vi "Gyro Vision Update.vi"() -> ()   [LabVIEW 2013]
uses:
  Robot Global Data.vi
  <vilib>/Rock Robotics/WPI/Gyro/WPI_GyroRefNum Registry Get.vi
  <vilib>/Rock Robotics/WPI/Gyro/WPI_GyroGetAngle.vi
panel:
  out "Success":bool
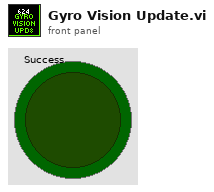
[diagram p1: front panel]
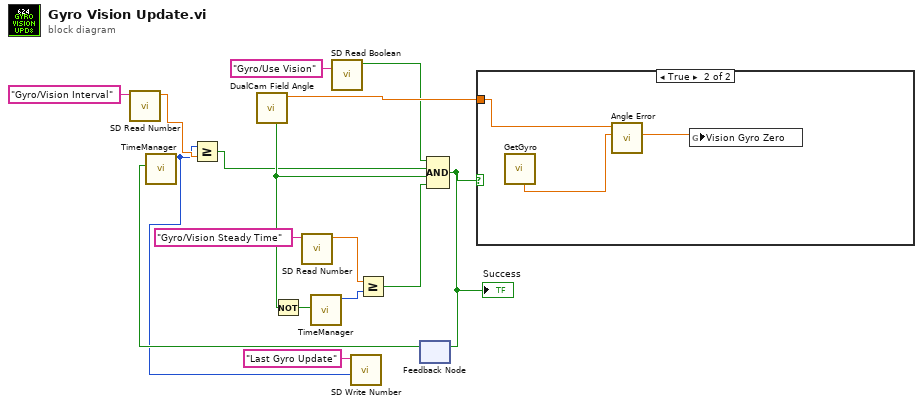
[diagram p0: block diagram]
diagram:
  n1 = call <vilib>:"SD Read Number.vi"("Name"="Gyro/Vision Interval") -> ("Numeric"=w8:dbl)  [unwired: 8 in, 2 out]
  n2 = call "DualCam Field Angle.vi"() -> ("Gyro Angle"=w16:dbl, "Found?"=w10:bool)  [unwired: 8 in, 2 out]
  n3 = Not(x=w10) -> (.not. x?=w15:bool)
  n4 = call <vilib>:"SD Read Number.vi"("Name"="Gyro/Vision Steady Time") -> ("Numeric"=w13:dbl)  [unwired: 8 in, 2 out]
  n5 = call "TimeManager.vi"("Reset?"=w15) -> ("Time Since Reset"=w12:u32)  [unwired: 9 in, 1 out]
  n6 = call <vilib>:"SD Read Boolean.vi"("Name"="Gyro/Use Vision") -> ("Boolean"=w1:bool)  [unwired: 8 in, 2 out]
  n7 = Greater Or Equal?(x=w13, y=w12) -> (x >= y?=w11:bool)
  n8 = feedback #1() -> (w6:bool)  [unwired: 1 in]
  n9 = call "TimeManager.vi"("Reset?"=w6) -> ("Time Since Reset"=w3:u32)  [unwired: 9 in, 1 out]
  n10 = Greater Or Equal?(x=w3, y=w8) -> (x >= y?=w7:bool)
  n11 = call <vilib>:"SD Write Number.vi"("Numeric"=w3, "Name"="Last Gyro Update") -> ()  [unwired: 8 in, 2 out]
  n12 = Compound Arithmetic op=AND(w1, w7, w10, w11) -> (w5:bool)
  "Success" <- w5
  n13 = feedback-in #1(w5) -> ()
  n14 = case shown="True" w5 {
    tunnel: w16 -> [_ w19]
    frame False {
    }
    frame True {
      n15 = call "GetGyro.vi"() -> ("Raw Angle"=w18:dbl)  [unwired: 9 in, 2 out]
      n16 = call "Angle Error.vi"("Angle"=w18, "Target Angle"=w19) -> ("Error"=w17:dbl)  [unwired: 9 in]
      n17 = global write "Robot Global Data.vi" "Vision Gyro Zero"(w17) -> ()
    }
  }
